vi "load new firmware.vi"(8 "error in (no error)":errorcluster, 9 "board_num":u16, 10 "filename":string, 11 "identifier":string) -> (0 "error out":errorcluster, 2 "filename out":string, 3 "function return":u32)   [LabVIEW 2015, in "XGL_DPP.lvlib"]
doc: "EXTERN DECLSPEC uint32_t CALL_CONV load_new_firmware(const char * identifier, char * filename, uint16_t board_num);"
uses:
  XGL_DPP.lvlib
  XGL_DPP.dll
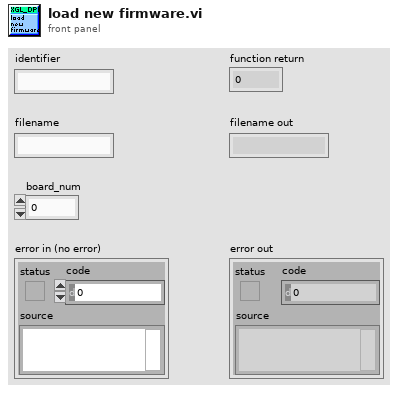
[diagram p1: front panel]
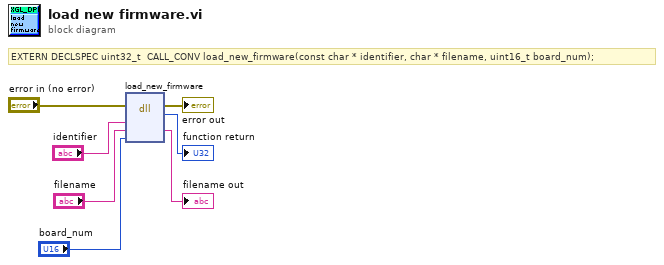
[diagram p0: block diagram]
diagram:
  # "EXTERN DECLSPEC uint32_t  CALL_CONV load_new_firmware(const char * identifier, char * filename, uint16_t board_num);"
  n1 = dll-call lib="D:/Users/XRF/Desktop/Scanning Software_Demokritos_2015_v7/libs/Vis_2/XGL_DPP.*" fn="load_new_firmware"(error in="error in (no error)", "identifier"="identifier", "filename"="filename", "board_num"="board_num") -> (error out=→"error out":errorcluster, →"function return":u32, "filename"=→"filename out":string)  [unwired: 4 in, 1 out]
